vi "Generate Name-Value Pair Array.vi"(11 "Name-Value Pair JSON":string) -> (3 "Name-Value Pairs":T1[](array[typedef]))   [LabVIEW 2015, in "NI_JSON Parsing.lvlib"]
uses:
  NI_JSON Parsing.lvlib
  Core/HTTP Request/Name Value Pair.ctl
  Core/HTTP Request/HTTP Request.lvclass
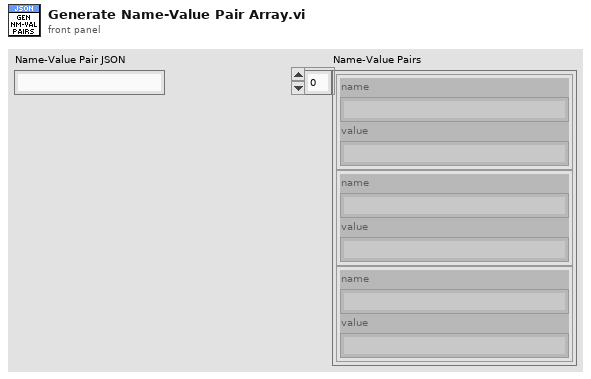
[diagram p1: front panel]
types:
  T1 = typedef "NI_AWS_Core.lvlib/HTTP Request.lvclass/Name Value Pair.ctl" = cluster{"name":string, "value":string}
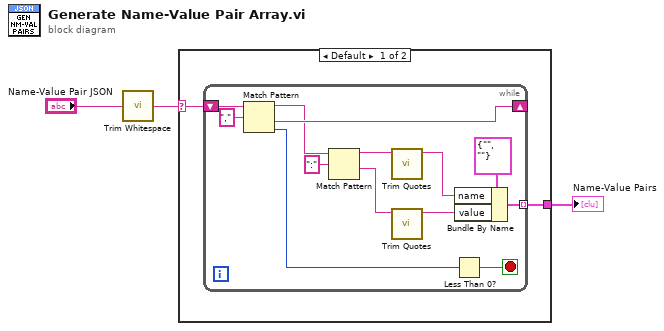
[diagram p0: block diagram]
diagram:
  n1 = call <vilib>:"Trim Whitespace.vi"("string"="Name-Value Pair JSON") -> ("trimmed string"=w1:string)  [unwired: 1 in]
  n2 = case shown="Default" w1 {
    selector: w1 -> [w4 _]
    tunnel: [w5 _] -> w2
    frame Default {
      n3 = while {
        shift-right: [w12] -> _
        shift-left: w4 -> [w18]
        tunnel: [w15] -> w5 mode=indexing
        stop <- w13 stop-if-true
        n4 = Match Pattern(string=w18, regular expression=",") -> (before substring=w11:string, after substring=w12:string, offset past match=w14:i32)  [unwired: 1 in, 1 out]
        n5 = Match Pattern(string=w11, regular expression=":" ("search string/char (-)")) -> (before substring=w9:string, after substring=w6:string)  [unwired: 1 in, 2 out]
        n6 = call "Trim Quotes.vi"("String"=w9) -> ("String without Quotes"=w8:string)  [unwired: 10 in]
        n7 = call "Trim Quotes.vi"("String"=w6) -> ("String without Quotes"=w7:string)  [unwired: 10 in]
        n8 = Less Than 0?(x=w14) -> (x < 0?=w13:bool)
        n9 = Bundle By Name(cluster=T1 {"name"="", "value"=""} ("Name Value Pair"), "name"=w8, "value"=w7) -> (w15:T1)
      }
    }
    frame "\u0000" {
    }
  }
  "Name-Value Pairs" <- w2
